vi "String to Base64-PORTABLE-5129.vi"(2 "Line separator (\\n)":string="\n", 7 "Plain String":string, 9 "error in":errorcluster) -> (8 "Base64 String":string, 10 "error out":errorcluster)   [LabVIEW 2020, in "Library Commun.lvlib"]
doc: "<inline>"
uses:
  Library Commun.lvlib
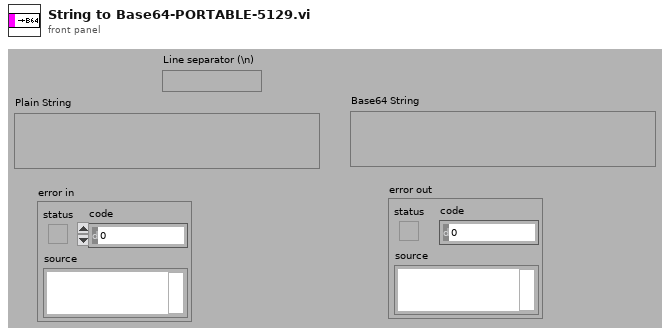
[diagram p1: front panel]
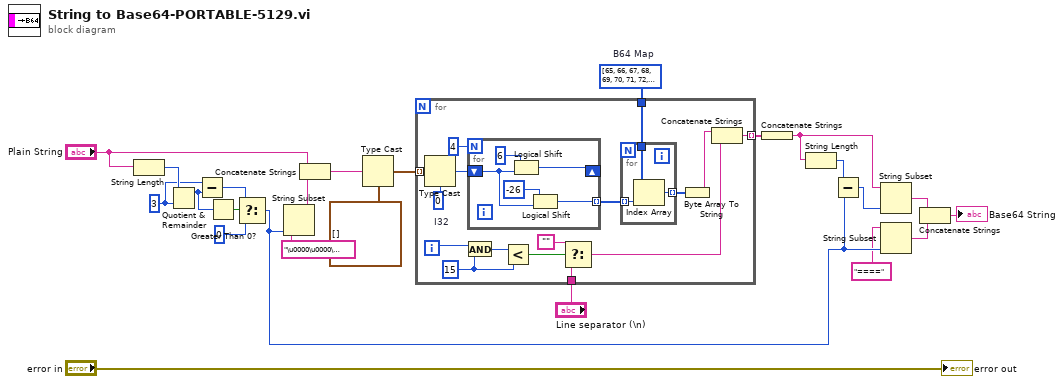
[diagram p0: block diagram]
diagram:
  w12 = u8[] [65, 66, 67, 68, 69, 70, 71, 72, 73, 74, 75, 76, 77, 78, 79, 80, 81, 82, 83, 84, 85, 86, 87, 88, 89, 90, 97, 98, 99, 100, 101, 102, 103, 104, 105, 106, 107, 108, 109, 110, 111, 112, 113, 114, 115, 116, 117, 118, 119, 120, 121, 122, 48, 49, 50, 51, 52, 53, 54, 55, 56, 57, 43, 47]  # B64 Map
  w18 = 3 ("y")
  n1 = String Length(string="Plain String") -> (length=w19:i32)
  n2 = Quotient & Remainder(x=w19, y=w18) -> (x-y*floor(x/y)=w17:i32)  [unwired: 1 out]
  n3 = Subtract(x=w18, y=w17) -> (x-y=w14:i32)
  n4 = Greater Than 0?(x=w17) -> (x > 0?=w16:bool)
  n5 = Select(t=w14, s=w16, f=0 ("y")) -> (s? t:f=w9:i32)
  n6 = String Subset(string="\u0000\u0000\u0000\u0000", length (rest)=w9) -> (substring=w23:string)  [unwired: 1 in]
  n7 = Concatenate Strings("Plain String", w23) -> (w21:string)
  n8 = Type Cast(type=cluster{"u8":u8, "u8":u8, "u8":u8}[] [], x=w21) -> (*(type *) &x=w13:cluster{"u8":u8, "u8":u8, "u8":u8}[])
  n9 = for {
    tunnel: w13 -> [w40] mode=indexing
    tunnel: w12 -> [w34]
    tunnel: "Line separator (\\n)" -> [w27]
    tunnel: [w25] -> w3 mode=indexing
    i -> [w30]
    w31 = 15 ("x")
    w39 = 0  # I32
    n10 = Type Cast(type=w39, x=w40) -> (*(type *) &x=w38:i32)
    n11 = And(x=w30, y=w31) -> (x .and. y?=w32:i32)
    n12 = for {
      N: 4 -> [_]
      shift-right: [w48] -> _
      shift-left: w38 -> [w45]
      tunnel: [w44] -> w35 mode=indexing
      n13 = Logical Shift(y=6, x=w45) -> (x << y=w48:i32)
      n14 = Logical Shift(y=-26, x=w45) -> (x << y=w44:i32)
    }
    n15 = Less?(x=w32, y=w31) -> (x < y?=w29:bool)
    n16 = Select(t="", s=w29, f=w27) -> (s? t:f=w26:string)
    n17 = for {
      tunnel: w35 -> [w43] mode=indexing
      tunnel: w34 -> [w42]
      tunnel: [w41] -> w33 mode=indexing
      n18 = Index Array(array=w42, index=w43) -> (element=w41:u8)
    }
    n19 = Byte Array To String(unsigned byte array=w33) -> (string=w37:string)
    n20 = Concatenate Strings(w37, w26) -> (w25:string)
  }
  n21 = Concatenate Strings(w3) -> (w2:string)
  n22 = String Length(string=w2) -> (length=w11:i32)
  n23 = Subtract(x=w11, y=w9) -> (x-y=w10:i32)
  n24 = String Subset(string=w2, length (rest)=w10) -> (substring=w7:string)  [unwired: 1 in]
  n25 = String Subset(string="====", length (rest)=w9) -> (substring=w6:string)  [unwired: 1 in]
  n26 = Concatenate Strings(w7, w6) -> (→"Base64 String":string)
  "error out" <- "error in"
